vi "CheckCancel.vi"(0 "error in (no error)":errorcluster) -> (1 "Cancelled":bool, 3 "error out":errorcluster)   [LabVIEW 2021]
uses:
  Globals and TypeDefs/Error Categories.ctt
  Globals and TypeDefs/gGeneral.vi
panel:
  out "call chain":string[](array[string])
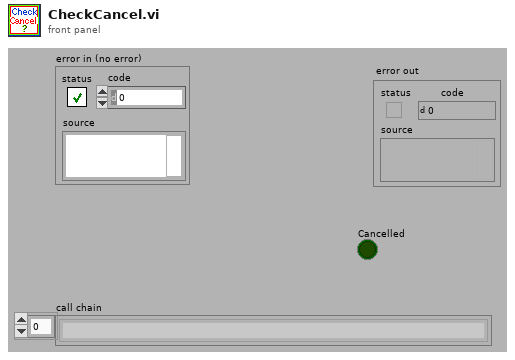
[diagram p1: front panel]
types:
  T1 = enum8{"Initialization Error", "Command Error", "Parameter Error", "Overflow Error", "Time-out Error", "Misc Error", "User cancel"}
  T2 = typedef "Error Categories.ctt" = enum8{"General", "CCD-256x1024", "CCD-1340x400", "InGaAs PDA", "McPherson 2075", "Magnetic Field", "Temperature Control", "Other"}
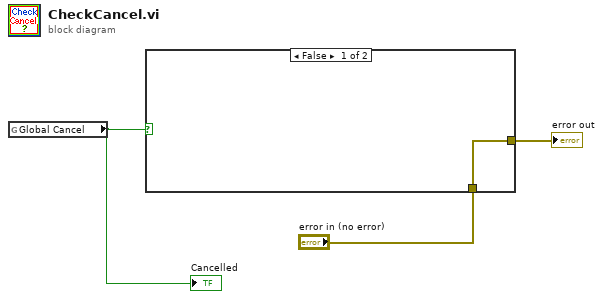
[diagram p0: block diagram]
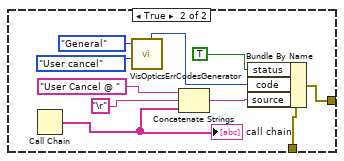
[diagram p2: hidden frame]
diagram:
  n1 = global read "gGeneral.vi" "Global Cancel"() -> (w1:bool)
  "Cancelled" <- w1
  n2 = case shown="False" w1 {
    tunnel: [w4 w14] -> w3
    tunnel: "error in (no error)" -> [w4 w5]
    frame False {
    }
    frame True {
      n3 = Call Chain() -> (call chain=w9:string[])
      "call chain" <- w9
      n4 = call "VisOpticsErrCodesGenerator.vi"("NHMFL Visible Optics Error Type"=T1."User cancel", "NHMFL Visible Optics Error Categories"=Error_Categories.ctt."General") -> ("User-defined Error Code"=w6:i32)  [unwired: 1 in, 5 out]
      n5 = Concatenate Strings("User Cancel @ " ("source"), "\r", w9) -> (w10:string)
      n6 = Bundle By Name(cluster=w5, "status"=TRUE, "code"=w6, "source"=w10) -> (w14:errorcluster)
    }
  }
  "error out" <- w3
